vi "XML - Get relative Configuration LLB path.vi"(8 "error in (no error)":errorcluster, 11 "CD Wizard - Internal Data":T1) -> (0 "error out":errorcluster, 3 "Relative Configuration LLB path":path)   [LabVIEW 2015]
doc: "Create the relative path for the Configuration LLB based on the name and execution mode of the new custom device."
uses:
  TypDef/CD Wizard - Internal data.ctl
  TypDef/CD Wizard - Execution Mode.ctl
  TypDef/CD Wizard - Extra Page Name and GUID.ctl
  Constants/Constants TypDef/Build Spec System Explorer.ctl
  Constants/Build Spec System Explorer.vi
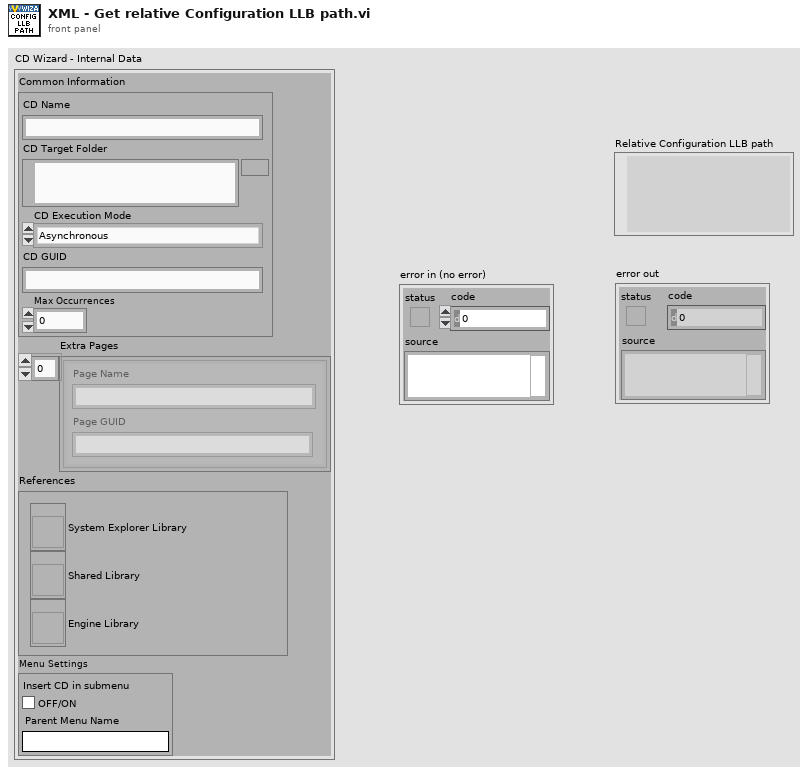
[diagram p1: front panel]
types:
  T1 = typedef "CD Wizard - Internal data.ctl" = cluster{"Common Information":cluster{"CD Name":string, "CD Target Folder":path, "CD Execution Mode":T2, "CD GUID":string, "Max Occurrences":u32}, "Extra Pages":T3[], "References":cluster{"System Explorer Library":refnum<vi>, "Shared Library":refnum<vi>, "Engine Library":refnum<vi>}, "Menu Settings":cluster{"Insert CD in submenu":bool, "Parent Menu Name":string}}
  T2 = typedef "CD Wizard - Execution Mode.ctl" = enum16{"Asynchronous", "Inline HW Interface", "Inline Model Interface", "Inline Timing and Sync", "Asynchronous Timing and Sync"}
  T3 = typedef "CD Wizard - Extra Page Name and GUID.ctl" = cluster{"Page Name":string, "Page GUID":string}
  T4 = typedef "Build Spec System Explorer.ctl" = enum16{"Destinations.LLBFileName"}
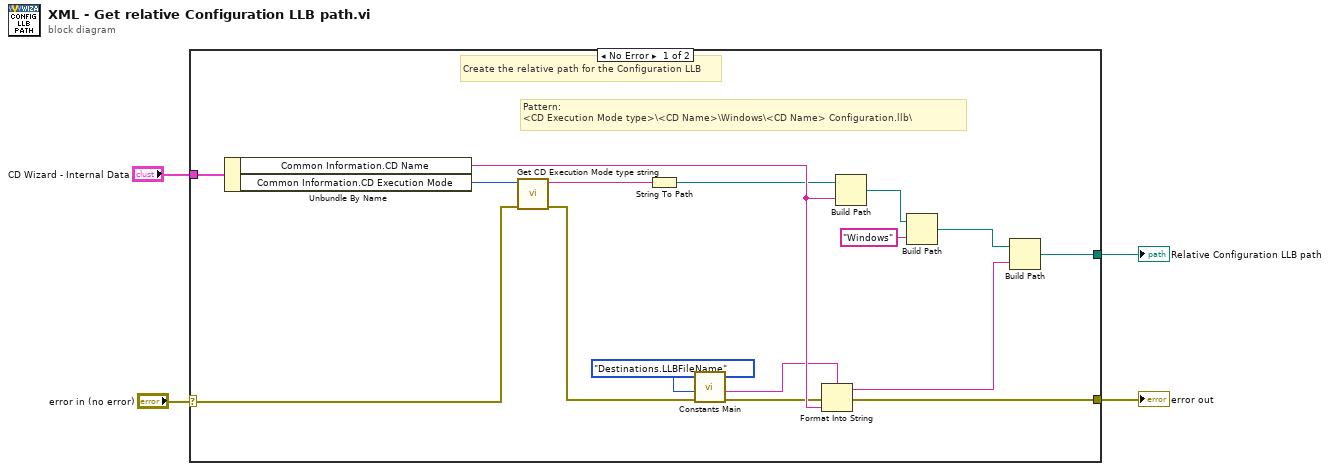
[diagram p0: block diagram]
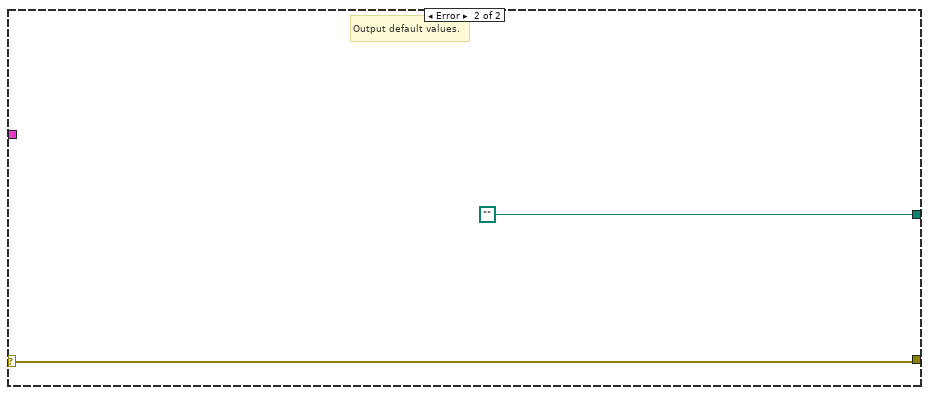
[diagram p2: hidden frame]
diagram:
  n1 = case shown="No Error" "error in (no error)" {
    selector: "error in (no error)" -> [w8 w22]
    tunnel: [w13 w22] -> w3
    tunnel: [w12 path ""] -> w1
    tunnel: "CD Wizard - Internal Data" -> [w14 _]
    frame No Error {
      # "Pattern:\n<CD Execution Mode type>\\<CD Name>\\Windows\\<CD Name> Configuration.llb\\"
      # "Create the relative path for the Configuration LLB"
      n2 = Unbundle By Name(w14) -> ("Common Information.CD Name"=w20:string, "Common Information.CD Execution Mode"=w10:T2)
      n3 = call "Get CD Execution Mode type string.vi"("error in (no error)"=w8, "CD Execution Mode"=w10) -> ("error out"=w9:errorcluster, "Execution Mode type"=w11:string)  [unwired: 8 in]
      n4 = String To Path(string=w11) -> (path=w15:path)
      n5 = call-poly "Constants Main.vi"("error in (no error)"=w9, "Action"=Build_Spec_System_Explorer."Destinations.LLBFileName") -> ("error out"=w17:errorcluster, "Output"=w18:string)  [unwired: 8 in]
      n6 = Format Into String(format string=w18, error in=w17, w20) -> (resulting string=w19:string, error out=w13:errorcluster)  [unwired: 1 in]
      n7 = Build Path(base path=w15, name or relative path=w20) -> (appended path=w7:path)
      n8 = Build Path(base path=w7, name or relative path="Windows") -> (appended path=w5:path)
      n9 = Build Path(base path=w5, name or relative path=w19) -> (appended path=w12:path)
    }
    frame Error {
      # "Output default values."
    }
  }
  "error out" <- w3
  "Relative Configuration LLB path" <- w1
